vi "Simulate Square Signal.vi"(8 "error in (no error)":errorcluster) -> (0 "error out":errorcluster, 3 "Square with Uniform Noise":dynamicdata(graph))   [LabVIEW 2023, in "Scope Simulated CFGs.lvlib" / "Fetch Waveforms CFG.lvclass"]
uses:
  Fetch Waveforms CFG.lvclass
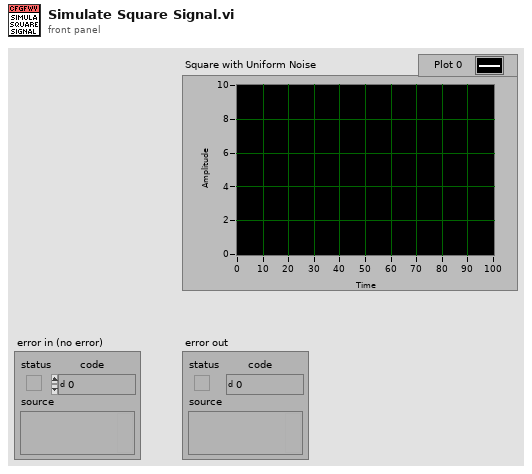
[diagram p1: front panel]
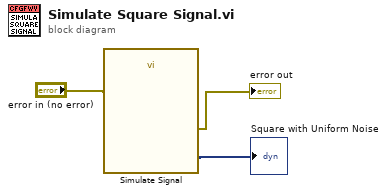
[diagram p0: block diagram]
diagram:
  n1 = call "Simulate Signal"("error in (no error)"="error in (no error)") -> ("Square with Uniform Noise"=→"Square with Uniform Noise":dynamicdata, "error out"=→"error out":errorcluster)  [unwired: 13 in]
